vi "COMI US Retrv Block.vi"(7 "VarType":u32(ring) items=["VT_SHORT", "VT_FLOAT", "VT_DOUBLE"], 9 "maxNumScan":i32, 10 "startCount":u32, 11 "hDevice":u32) -> (2 "function return":u32, 3 "hDevice out":u32)   [LabVIEW 2017, in "Comidll.lvlib"]
doc: "unsigned int (COMI_US_RetrvBlock) (HANDLE hDevice, unsigned int startCount, int maxNumScan, \n void pDestBuf, TComiVarType VarType);"
uses:
  <userlib>/Comidll/Comidll.lvlib
  <userlib>/Comidll/Comidll.dll
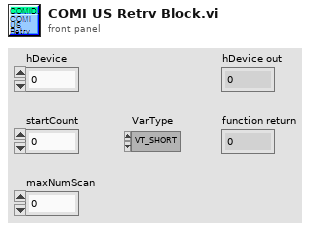
[diagram p1: front panel]
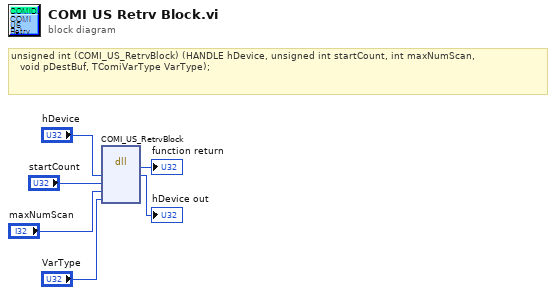
[diagram p0: block diagram]
diagram:
  # "unsigned int\t(COMI_US_RetrvBlock) (HANDLE hDevice, unsigned int startCount, int maxNumScan, \n\t\t\tvoid pDestBuf, TComiVarType VarType);"
  n1 = dll-call lib="C:/Program Files/National Instruments/LabVIEW 2017/user.lib/Comidll/Comidll.*" fn="COMI_US_RetrvBlock"("hDevice"="hDevice", "startCount"="startCount", "maxNumScan"="maxNumScan", "VarType"="VarType") -> (→"function return":u32, "hDevice"=→"hDevice out":u32)  [unwired: 6 in, 2 out]
